vi "Gewinner(SubVI).vi"(10 "Array":u8[][](array[numeric]), 11 "Next Turn":i8) -> (1 "Game over":bool, 2 "Win 2":bool, 3 "Win":bool)   [LabVIEW 2017]
uses:
  Opponent.vi
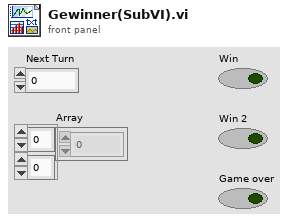
[diagram p1: front panel]
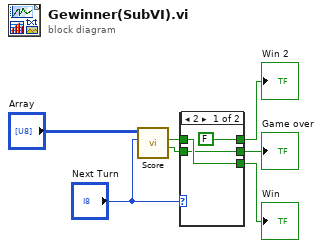
[diagram p0: block diagram]
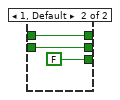
[diagram p2: hidden frame]
diagram:
  n1 = call "Score.vi"("SpielerZuege"="Next Turn", "Game"="Array") -> ("Game over"=w7:bool, "Win"=w3:bool)  [unwired: 7 in, 1 out]
  n2 = case shown="2" "Next Turn" {
    tunnel: [FALSE w13] -> w1
    tunnel: w3 -> [w9 w13]
    tunnel: [w9 FALSE] -> w2
    tunnel: w7 -> [w8 w11]
    tunnel: [w8 w11] -> w4
    frame 2 {
    }
    frame 1, Default {
    }
  }
  "Game over" <- w4
  "Win" <- w2
  "Win 2" <- w1
